vi "SaveData.vi"(8 "error in (no error)":errorcluster, 10 "PrintNum":u16 caption="列印數:", 11 "Data In":T1) -> (0 "error out":errorcluster, 3 "Data Out":T1)   [LabVIEW 2014]
uses:
  controls/Data1.ctl
  controls/Payjson.ctl
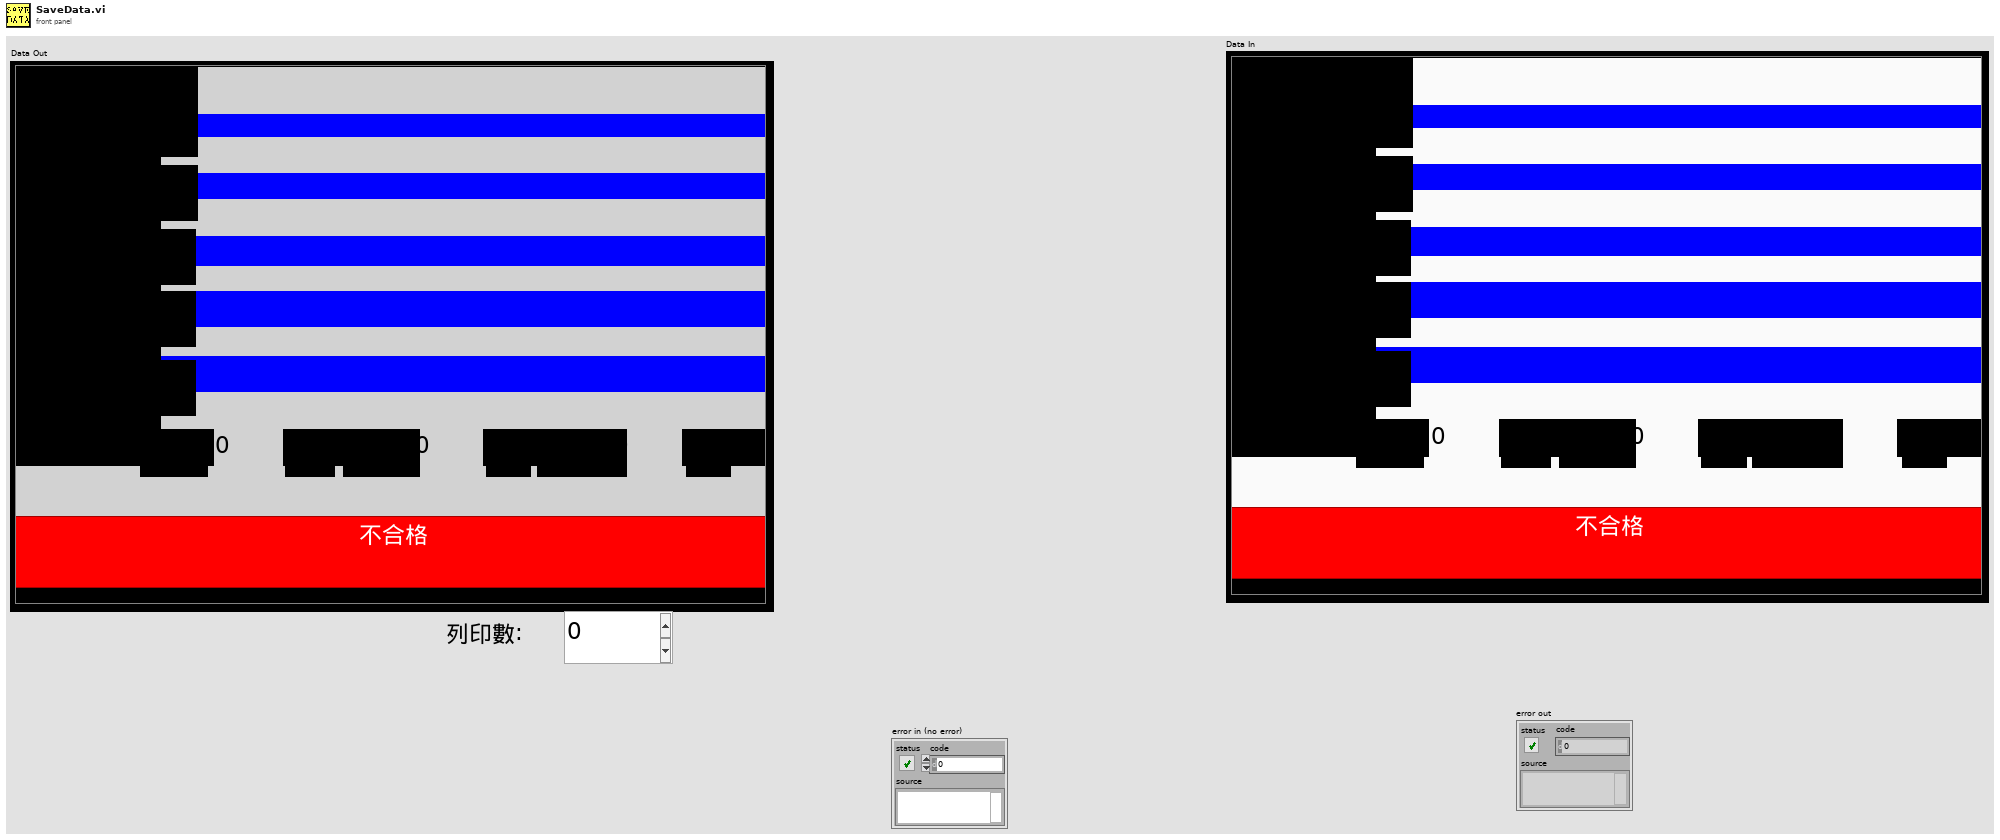
[diagram p1: front panel]
types:
  T1 = typedef "Data1.ctl" = cluster{"Date":string, "BarCode1":string, "BarCode2":string, "BarCode3":string, "Message":string, "OK Count":u16, "NG Count":u16, "Total Count":u16, "ModelData":string[][], "OK&NG":bool, "COM1":refnum<visa-resource-name>, "COM2":refnum<visa-resource-name>, "IO":i32, "Time":u32, "TCP":refnum<k5>, "TCP 2":refnum<k5>, "COM1 2":refnum<visa-resource-name>, "CheckNum":string, "BarCode1_1":string, "BarCode2_1":string, "BarCode3_1":string, "日期":string, "機種":string, "機號":string, "商品條碼1":string, "OK_1":string, "OK":string, "NG":string, "NG_1":string, "Total":string, "Total_1":string, "ClaerTime":u32, "Pjson":T2, "LotNo":string[], "CheckParsArray":string[], "BarCode4":string, "BarCode4_1":string, "商品條碼2":string, "BarCode5":string, "BarCode5_1":string, "商品條碼3":string, "ReScanNG":i32, "NGTimeCT":u32}
  T2 = typedef "Payjson.ctl" = cluster{"DEPT":string, "LINE":string, "STANO":string, "WORKNO":string, "PRODSN":string, "COMPNTID":string, "COMPNTLOT":string, "COMPNTSN":string, "USEDQTY":i16, "OPDATE":string, "OPUSER":string, "RECVDATE":string, "MMODU":string}[]
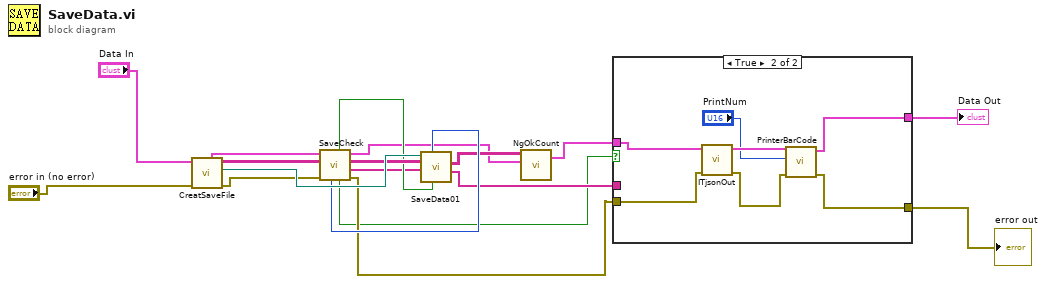
[diagram p0: block diagram]
diagram:
  n1 = call "CreatSaveFile.vi"("error in (no error)"="error in (no error)", "Data_In"="Data In") -> ("error out"=w7:errorcluster, "FileSave path"=w17:path, "DataTable"=w18:string[][], "Data_out"=w2:T1)  [unwired: 6 in]
  n2 = call "SaveCheck.vi"("error in (no error)"=w7, "DataTable In"=w18, "Data In"=w2) -> ("error out"=w6:errorcluster, "Save Data"=w14:string[], "DataTable Out"=w16:string[][], "Data Out"=w11:T1, "IT Save?"=w1:bool, "Dupicate"=w15:bool, "index (row)"=w13:i32)  [unwired: 2 in]
  n3 = call "SaveData01.vi"("Dupicate"=w15, "Index Row"=w13, "Save Data In"=w14, "DataTable In"=w16, "file path (dialog if empty)"=w17) -> ("Save Data Out"=w10:string[], "DataTable Out"=w12:string[][])  [unwired: 5 in]
  n4 = call "NgOkCount.vi"("Data In"=w11, "Data Table In"=w12) -> ("Data Out"=w5:T1)  [unwired: 5 in, 4 out]
  n5 = case shown="True" w1 {
    tunnel: w10 -> [_ _]
    tunnel: w6 -> [w20 w26]
    tunnel: [w20 w23] -> w9
    tunnel: w5 -> [w19 w27]
    tunnel: [w19 w22] -> w4
    frame False {
    }
    frame True {
      n6 = call "ITjsonOut.vi"("error in (no error)"=w26, "Data In"=w27) -> ("error out"=w24:errorcluster, "Data Out"=w25:T1)  [unwired: 8 in]
      n7 = call "PrinterBarCode.vi"("error in (no error)"=w24, "PrintNum"="PrintNum", "Data In"=w25) -> ("error out"=w23:errorcluster, "Data Out"=w22:T1)  [unwired: 7 in]
    }
  }
  "Data Out" <- w4
  "error out" <- w9
